vi "Teleop.vi"(10 "Match Info":T2={"Autonomous Elapsed Seconds"=0.0, "TeleOp Elapsed Seconds"=0.0, "Disabled Elapsed Seconds"=0.0, "Visited Autonomous"=FALSE, "Visited TeleOp"=FALSE, "Visited Disabled"=FALSE, "Autonomous Settings"={"Autonomous Style"=enum."Independent", "VI Refnum"=refnum}}, 11 "Call Context":T3) -> ()   [LabVIEW 2012]
doc: "This VI is called for each TeleOp packet received from the DS where the robot is not disabled. It is often used to read from the joysticks and update I/O or to update setpoints for timed control loops. It should complete and return within 20 milliseconds or it may miss DS packets."
uses:
  <vilib>/Rock Robotics/WPI/DriverStation/WPI_DriverStationDerivedRobotMode.ctl
  <vilib>/Rock Robotics/WPI/DriverStation/WPI_DriverStationMatch Info.ctl
  <vilib>/Rock Robotics/WPI/Relay/WPI_RelayValue.ctl
  <vilib>/Rock Robotics/WPI/Solenoid/WPI_SolenoidValue.ctl
  Robot Global Data.vi
  <vilib>/addons/control/pid/pid.llb/PID (DBL).vi
  <vilib>/Rock Robotics/WPI/RobotDrive/WPI_RobotDriveGetSetRefNum.vi
  <vilib>/Rock Robotics/WPI/Joystick/WPI_JoystickGetSetRefNum.vi
  <vilib>/Rock Robotics/WPI/Solenoid/WPI_SolenoidSetEnum.vi
  <vilib>/addons/control/pid/NI_PID_pid.lvlib
panel:
  in  "Boolean":bool
  in  "Time to twitch":dbl=1300.0
  in  "Time of start twitch":dbl
  in  "Turn speed for twitch":dbl=0.7
  in  "Twitch":string="Nope"
  in  "Threshold for shooter":dbl=0.015
  in  "Posistioned":string="Nothing"
  in  "Angle Target":dbl
  out "Distance From Target":dbl
  out "Ready To Fire":bool
  in  "S Off Time":dbl=1.2
  in  "S On Time":dbl=0.2
  in  "Time Last Fired":dbl
  in  "Current Status":string="Roaming"
  in  "Shooter Speed":dbl format="%.2f"
  in  "Shooter On":bool=TRUE
  out "Waveform Chart":cluster{"Rate":dbl, "Rate":dbl}(graph)
  out "Rate 1":dbl
  out "Rate 2":dbl
  in  "PID gains":T1={"proportional gain (Kc)"=1.0, "integral time (Ti, min)"=0.007, "derivative time (Td, min)"=0.0} {"derivative time (Td, min)" format="%.3f"; "integral time (Ti, min)" format="%.3f"; "proportional gain (Kc)" format="%.3f"}
  in  "Maximum Encoder speed":dbl=25000.0
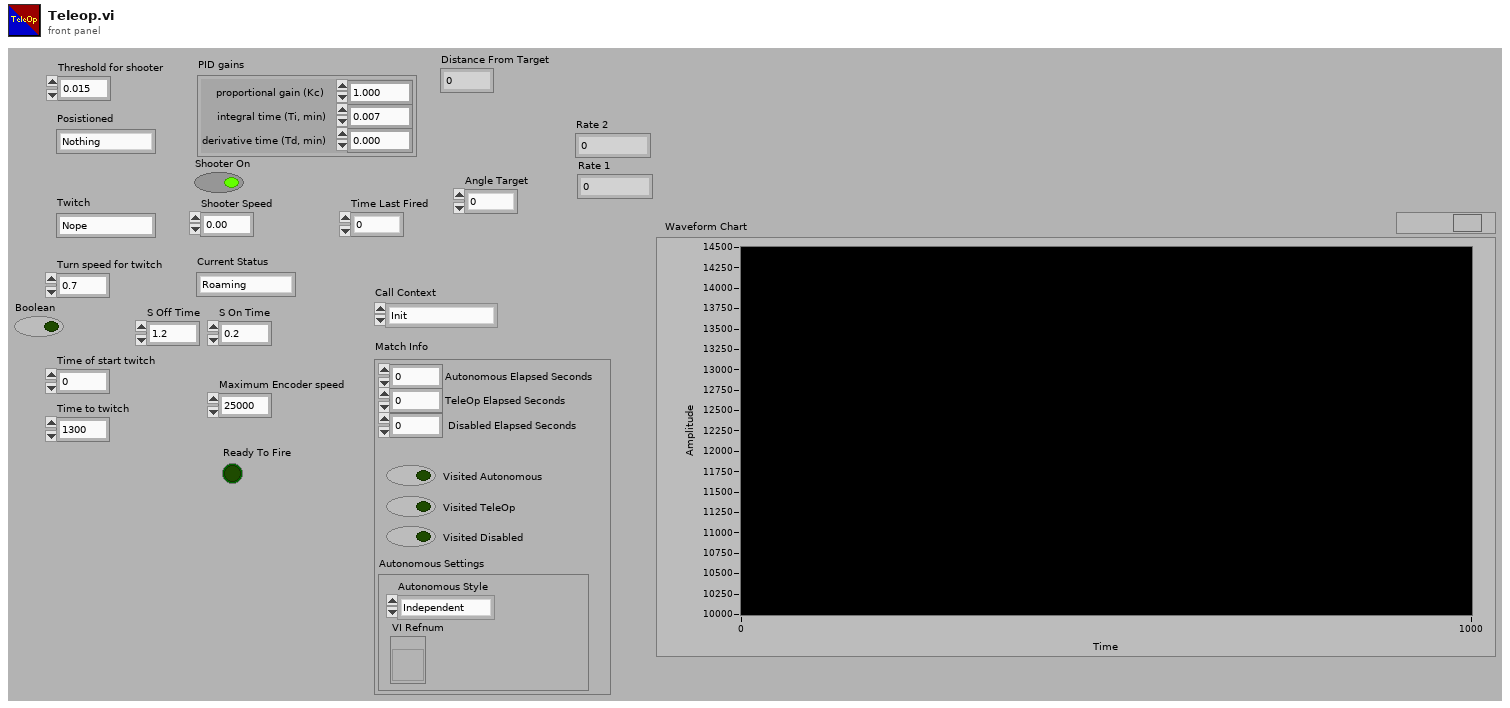
[diagram p1: front panel]
types:
  T1 = cluster{"proportional gain (Kc)":dbl, "integral time (Ti, min)":dbl, "derivative time (Td, min)":dbl}
  T2 = typedef "WPI_DriverStationMatch Info.ctl" = cluster{"Autonomous Elapsed Seconds":dbl, "TeleOp Elapsed Seconds":dbl, "Disabled Elapsed Seconds":dbl, "Visited Autonomous":bool, "Visited TeleOp":bool, "Visited Disabled":bool, "Autonomous Settings":cluster{"Autonomous Style":enum16{"Iterative", "Independent"}, "VI Refnum":refnum<vi>}}
  T3 = typedef "WPI_DriverStationDerivedRobotMode.ctl" = enum16{"Init", "Execute", "Stop"}
  T4 = typedef "WPI_EncoderDevRef.ctl" = cluster{"DevStatus":errorcluster, "EncoderIndex":T5, "CounterIndex":T6, "DistancePerCount":dbl, "Decoding Type":T7}
  T5 = typedef "FPGA_EncoderIdx.ctl" = enum8{"Enc 0", "Enc 1", "Enc 2", "Enc 3", "Invalid"}
  T6 = typedef "FPGA_CounterCtrSystemIndex.ctl" = enum8{"Ctr 0", "Ctr 1", "Ctr 2", "Ctr 3", "Ctr 4", "Ctr 5", "Ctr 6", "Ctr 7", "Invalid"}
  T7 = typedef "WPI_EncoderType.ctl" = enum16{"1x", "2x", "4x"}
  T8 = typedef "WPI_JoystickDevRef.ctl" = cluster{"Device":T9}
  T9 = typedef "WPI_JoystickDeviceEnum.ctl" = enum16{"USB 1", "USB 2", "USB 3", "USB 4", "Kinect 1", "Kinect 2"}
  T10 = typedef "WPI_JoystickButtonState.ctl" = cluster{"Button 1":bool, "Button 2":bool, "Button 3":bool, "Button 4":bool, "Button 5":bool, "Button 6":bool, "Button 7":bool, "Button 8":bool, "Button 9":bool, "Button 10":bool, "Button 11":bool, "Button 12":bool}
  T11 = cluster{"axis 1 (x)":dbl, "axis 2 (y)":dbl, "axis 3 (throttle)":dbl, "axis 4":dbl, "axis 5":dbl, "axis 6":dbl}
  T12 = typedef "WPI_RobotDriveDevRef.ctl" = cluster{"DevStatus":errorcluster, "Motors[]":T13[], "Square Inputs":bool, "Max Output":dbl, "Isochronous":bool}
  T13 = typedef "WPI_MotorControlDeviceRef.ctl" = cluster{"DeviceStatus":errorcluster, "Type":enum16{"PWM", "CAN"}, "PWM":cluster{"Digital Module":T14, "PWM Channel":T15, "DeadBand":T16}, "CAN":cluster{"Device Number":u8, "Control Mode":T17, "Semaphore":T18, "Max Vout":dbl}, "Invert":bool, "TransformRef":T19, "InvTransformRef":T19}
  T14 = typedef "FPGA_TypedefDigitalModule.ctl" = enum16{"Digital Module 1", "Digital Module 2"}
  T15 = typedef "FPGA_DIOPWMChannel.ctl" = enum8{"PWM 1", "PWM 2", "PWM 3", "PWM 4", "PWM 5", "PWM 6", "PWM 7", "PWM 8", "PWM 9", "PWM 10", "Invalid"}
  T16 = typedef "WPI_PWMDeadband.ctl" = cluster{"Name":string, "maxPositivePwm":i32, "minPositivePwm":i32, "centerPwm":i32, "maxNegativePwm":i32, "minNegativePwm":i32, "angularRange":u16}
  T17 = typedef "WPI_CANJaguar_ControlMode.ctl" = enum8{"Percent VBus", "Current", "Speed", "Position", "Voltage"}
  T18 = typedef "Semaphore RefNum" = refnum<k1>
  T19 = typedef "WPI_PWMTransform_ConPane.ctl" = refnum<vi>
  T20 = typedef "WPI_RelayValue.ctl" = enum16{"Off", "On", "Forward", "Reverse"}
  T21 = typedef "WPI_RelayDevRef.ctl" = cluster{"DevStatus":errorcluster, "Relay Channel":T22, "Digital Module":T14, "Relay Direction":T23}
  T22 = typedef "FPGA_DIORelayChannel.ctl" = enum8{"Relay 1", "Relay 2", "Relay 3", "Relay 4", "Relay 5", "Relay 6", "Relay 7", "Relay 8", "Invalid"}
  T23 = typedef "WPI_RelayDirection.ctl" = enum16{"Both directions", "Forward only", "Reverse only"}
  T24 = typedef "WPI_SolenoidValue.ctl" = enum16{"Off", "On", "Forward", "Reverse"}
  T25 = typedef "WPI_SolenoidDevRef.ctl" = cluster{"DevStatus":errorcluster, "Solenoid Module":T26, "Forward Solenoid Channel":T27, "Reverse Solenoid Channel":T27}
  T26 = typedef "FPGA_TypedefSolenoidModule.ctl" = enum16{"Solenoid Module 1", "Solenoid Module 2"}
  T27 = typedef "WPI_SolenoidChannel.ctl" = enum8{"Solenoid 1", "Solenoid 2", "Solenoid 3", "Solenoid 4", "Solenoid 5", "Solenoid 6", "Solenoid 7", "Solenoid 8", "Invalid"}
  T28 = cluster{"Center Position":cluster{"X":dbl, "Y":dbl}, "Distance (ft)":dbl, "Center":bool}[]
  T29 = cluster{"Center Position":cluster{"X":dbl, "Y":dbl}, "Distance (ft)":dbl, "Center":bool}
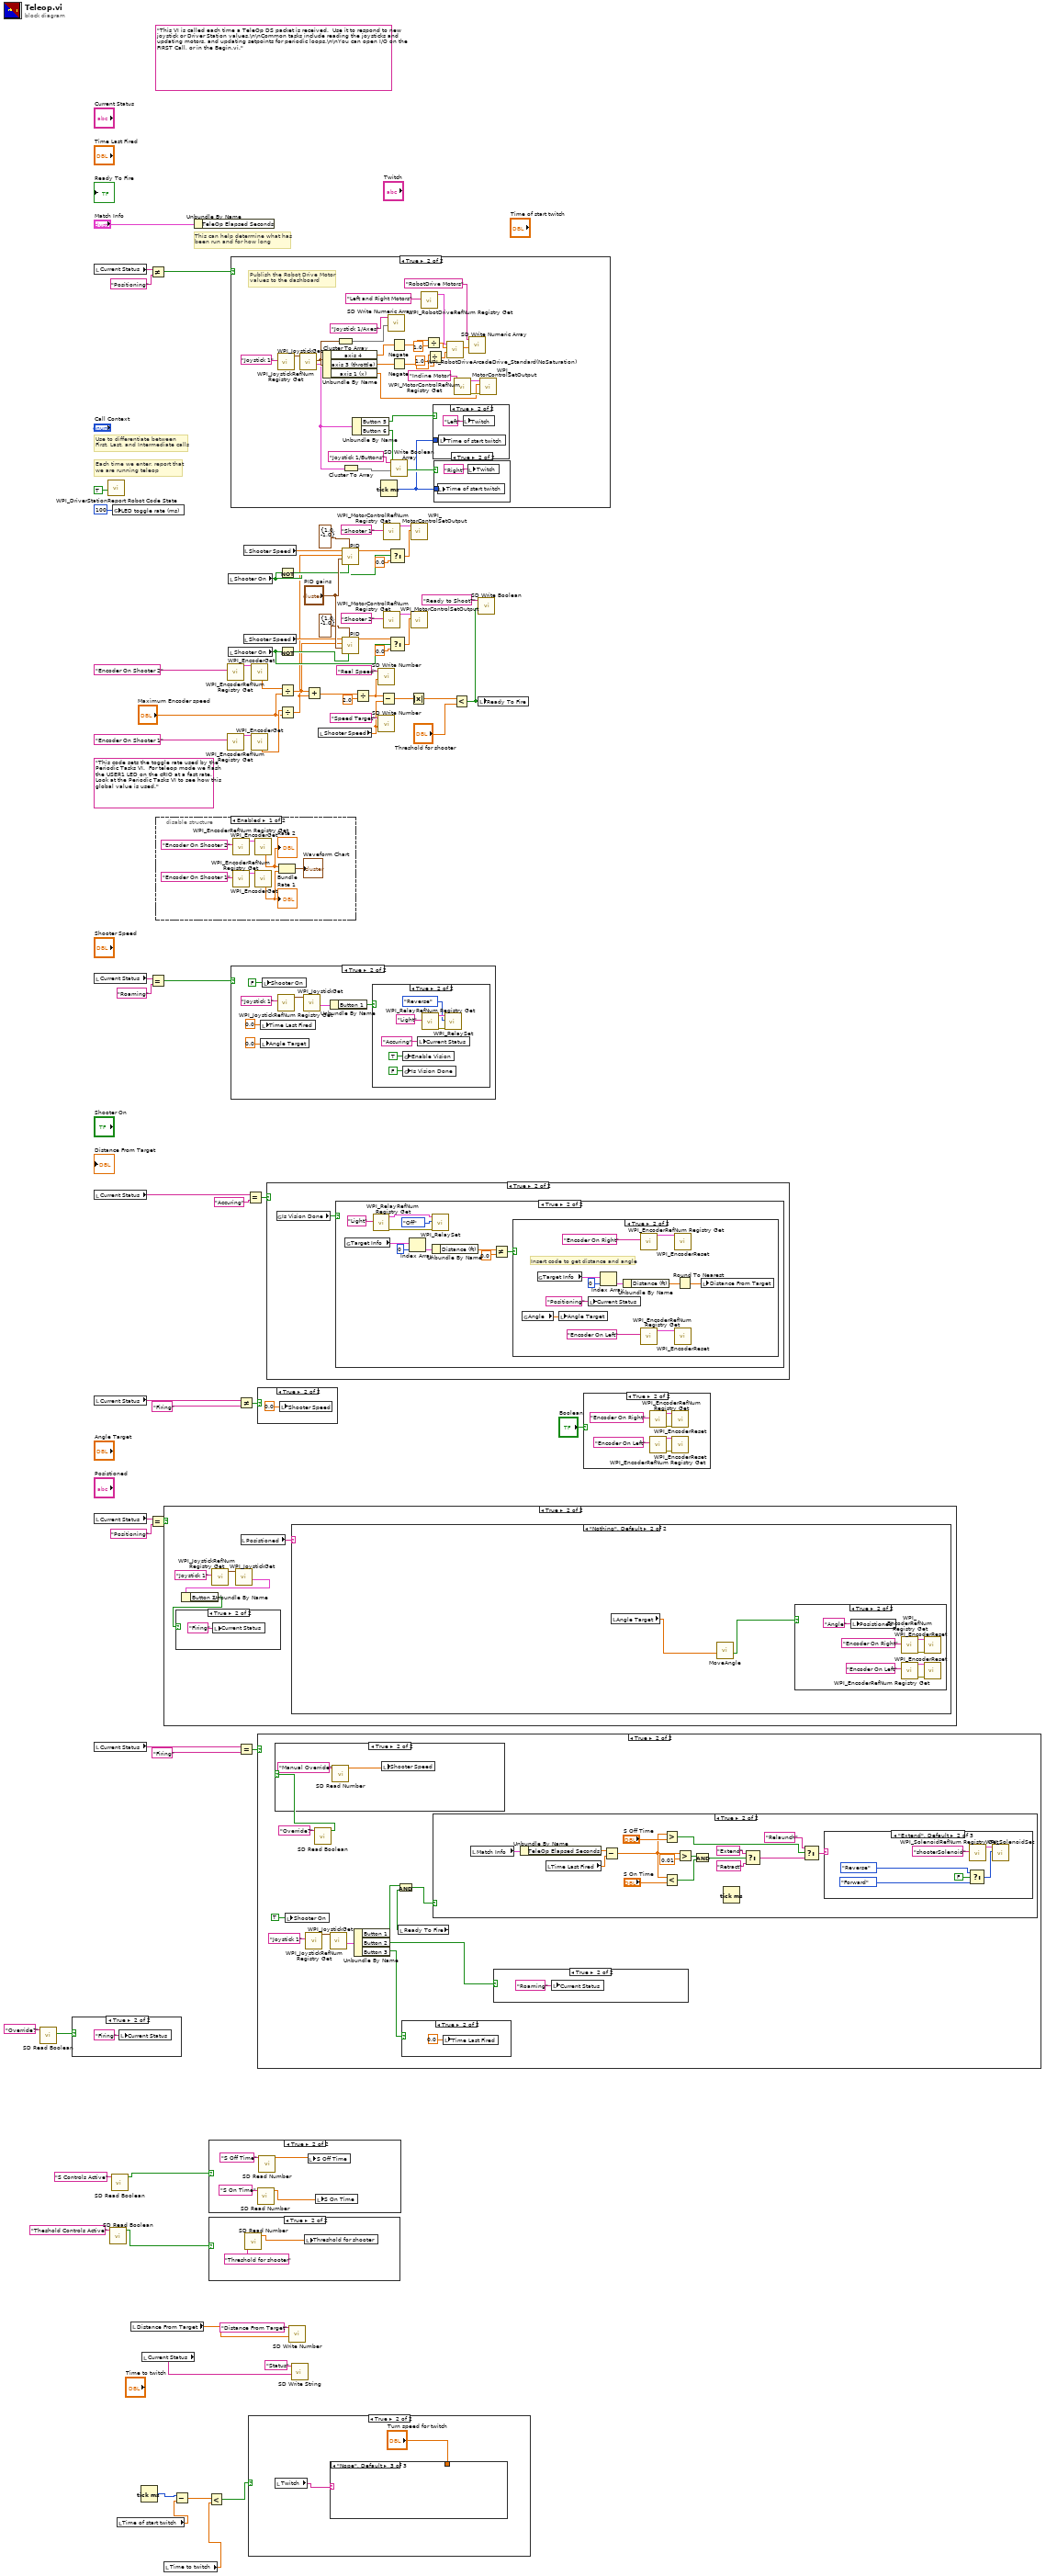
[diagram p0: block diagram]
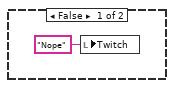
[diagram p3: hidden frame]
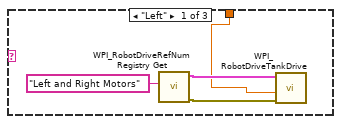
[diagram p4: hidden frame]
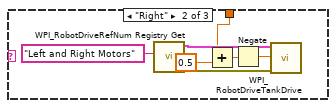
[diagram p5: hidden frame]
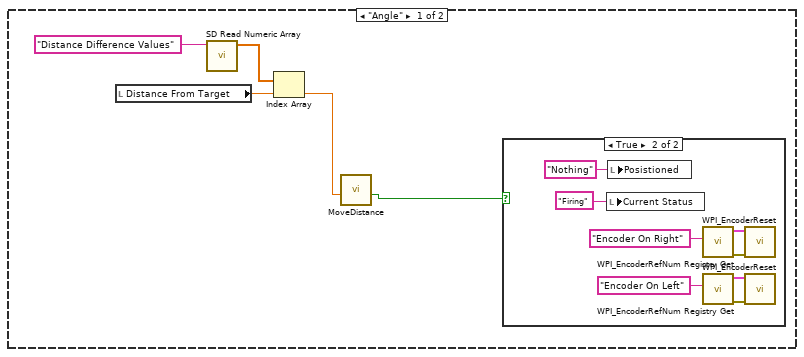
[diagram p12: hidden frame]
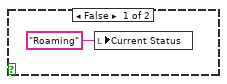
[diagram p20: hidden frame]
diagram:
  (unwired) "This code sets the toggle rate used by the Periodic Tasks VI.  For teleop mode we flash the USER1 LED on the cRIO at a fast rate.  Look at the Periodic Tasks VI to see how this global value is used."
  (unwired) "This VI is called each time a TeleOp DS packet is received.  Use it to respond to new joystick or Driver Station values.\n\nCommon tasks include reading the joysticks and updating motors, and updating setpoints for periodic loops.\n\nYou can open I/O on the FIRST Call, or in the Begin.vi."
  # "Each time we enter, report that\nwe are running teleop"
  # "Use to differentiate between\nFirst, Last, and Intermediate calls"
  # "This can help determine what has\nbeen run and for how long"
  n1 = call <vilib>:"SD Read Boolean.vi"("Name"="Override?") -> ("Boolean"=w15:bool)  [unwired: 8 in, 2 out]
  n2 = case shown="True" w15 {
    frame False {
    }
    frame True {
      n3 = local write "Current Status"("Firing" ("Current Status")) -> ()
    }
  }
  n4 = local read "Current Status"() -> (w26:string)
  n5 = local read "Current Status"() -> (w32:string)
  n6 = local read "Current Status"() -> (w29:string)
  n7 = local read "Current Status"() -> (w19:string)
  n8 = local read "Current Status"() -> (w23:string)
  n9 = local read "Current Status"() -> (w47:string)
  n10 = call <vilib>:"WPI_DriverStationReport Robot Code State.vi"("TeleOp"=TRUE ("Autonomous")) -> ()  [unwired: 10 in, 1 out]
  n11 = call <vilib>:"SD Read Boolean.vi"("Name"="Theshold Controls Active") -> ("Boolean"=w14:bool)  [unwired: 8 in, 2 out]
  n12 = call <vilib>:"SD Read Boolean.vi"("Name"="S Controls Active") -> ("Boolean"=w12:bool)  [unwired: 8 in, 2 out]
  n13 = global write "Robot Global Data.vi" "LED toggle rate (ms)"(u32 100 ("LED ms toggle rate")) -> ()
  n14 = local read "Time of start twitch"() -> (w6:dbl)
  n15 = local read "Distance From Target"() -> (w9:dbl)
  n16 = Tick Count (ms)() -> (millisecond timer value=w7:u32)
  n17 = local read "Current Status"() -> (w1:string)
  n18 = Not Equal?(x=w26, y="Positioning") -> (x != y?=w24:bool)
  n19 = Equal?(x=w32, y="Roaming") -> (x = y?=w30:bool)
  n20 = Equal?(x=w23, y="Positioning") -> (x = y?=w21:bool)
  n21 = disable-structure shown="Enabled" {
    frame Enabled {
      n22 = call <vilib>:"WPI_EncoderRefNum Registry Get.vi"("refnum name"="Encoder On Shooter 2") -> ("EncoderDevRef"=w83:T4)  [unwired: 9 in, 1 out]
      n23 = call <vilib>:"WPI_EncoderRefNum Registry Get.vi"("refnum name"="Encoder On Shooter 1") -> ("EncoderDevRef"=w82:T4)  [unwired: 9 in, 1 out]
      n24 = call <vilib>:"WPI_EncoderGet.vi"("EncoderDevRef"=w83) -> ("Rate"=w80:dbl)  [unwired: 5 in, 5 out]
      "Rate 2" <- w80
      n25 = call <vilib>:"WPI_EncoderGet.vi"("EncoderDevRef"=w82) -> ("Rate"=w81:dbl)  [unwired: 5 in, 5 out]
      "Rate 1" <- w81
      n26 = Bundle("Rate"=w80, "Rate"=w81) -> (→"Waveform Chart":cluster{"Rate":dbl, "Rate":dbl})  [unwired: 1 in]
    }
    frame Disabled {
    }
  }
  n27 = case shown="True" w21 {
    frame False {
    }
    frame True {
      n28 = call <vilib>:"WPI_JoystickRefNum Registry Get.vi"("refnum name"="Joystick 1") -> ("JoystickDevRef"=w87:T8)  [unwired: 9 in, 1 out]
      n29 = call <vilib>:"WPI_JoystickGet.vi"("JoystickDevRef"=w87) -> ("Buttons"=w86:T10)  [unwired: 4 in, 2 out]
      n30 = Unbundle By Name(w86) -> ("Button 2"=w85:bool)
      n31 = case shown="True" w85 {
        frame False {
        }
        frame True {
          n32 = local write "Current Status"("Firing" ("Current Status")) -> ()
        }
      }
      n33 = local read "Posistioned"() -> (w89:string)
      n34 = case shown="\"Nothing\", Default" w89 {
        frame "Angle" {
          n35 = local read "Distance From Target"() -> (w93:dbl)
          n36 = call <vilib>:"SD Read Numeric Array.vi"("Name"="Distance Difference Values") -> ("Numeric Array"=w95:dbl[])  [unwired: 8 in, 2 out]
          n37 = Index Array(array=w95, index=w93) -> (element=w92:dbl)
          n38 = call "MoveDistance.vi"("Distance From Target"=w92) -> ("Done?"=w91:bool)  [unwired: 10 in]
          n39 = case shown="True" w91 {
            frame False {
            }
            frame True {
              n40 = local write "Current Status"("Firing" ("Current Status")) -> ()
              n41 = local write "Posistioned"("Nothing" ("Posistioned")) -> ()
              n42 = call <vilib>:"WPI_EncoderRefNum Registry Get.vi"("refnum name"="Encoder On Right") -> ("error out"=w101:errorcluster, "EncoderDevRef"=w102:T4)  [unwired: 9 in]
              n43 = call <vilib>:"WPI_EncoderRefNum Registry Get.vi"("refnum name"="Encoder On Left") -> ("error out"=w99:errorcluster, "EncoderDevRef"=w100:T4)  [unwired: 9 in]
              n44 = call <vilib>:"WPI_EncoderReset.vi"("error in (no error)"=w101, "EncoderDevRef"=w102) -> ()  [unwired: 8 in, 2 out]
              n45 = call <vilib>:"WPI_EncoderReset.vi"("error in (no error)"=w99, "EncoderDevRef"=w100) -> ()  [unwired: 8 in, 2 out]
            }
          }
        }
        frame "Nothing", Default {
          n46 = local read "Angle Target"() -> (w105:dbl)
          n47 = call "MoveAngle.vi"("Angle Target"=w105) -> ("Done?"=w104:bool)  [unwired: 10 in]
          n48 = case shown="True" w104 {
            frame False {
            }
            frame True {
              n49 = local write "Posistioned"("Angle" ("Posistioned")) -> ()
              n50 = call <vilib>:"WPI_EncoderRefNum Registry Get.vi"("refnum name"="Encoder On Right") -> ("error out"=w108:errorcluster, "EncoderDevRef"=w107:T4)  [unwired: 9 in]
              n51 = call <vilib>:"WPI_EncoderRefNum Registry Get.vi"("refnum name"="Encoder On Left") -> ("error out"=w110:errorcluster, "EncoderDevRef"=w109:T4)  [unwired: 9 in]
              n52 = call <vilib>:"WPI_EncoderReset.vi"("error in (no error)"=w108, "EncoderDevRef"=w107) -> ()  [unwired: 8 in, 2 out]
              n53 = call <vilib>:"WPI_EncoderReset.vi"("error in (no error)"=w110, "EncoderDevRef"=w109) -> ()  [unwired: 8 in, 2 out]
            }
          }
        }
      }
    }
  }
  n54 = local read "Time to twitch"() -> (w4:dbl)
  n55 = Subtract(x=w7, y=w6) -> (x-y=w5:dbl)
  n56 = Unbundle By Name("Match Info") -> ()  [unwired: 1 out]
  n57 = Less?(x=w5, y=w4) -> (x < y?=w3:bool)
  n58 = case shown="True" w12 {
    frame False {
    }
    frame True {
      n59 = call <vilib>:"SD Read Number.vi"("Name"="S On Time") -> ("Numeric"=w115:dbl)  [unwired: 8 in, 2 out]
      n60 = call <vilib>:"SD Read Number.vi"("Name"="S Off Time") -> ("Numeric"=w116:dbl)  [unwired: 8 in, 2 out]
      n61 = local write "S Off Time"(w116) -> ()
      n62 = local write "S On Time"(w115) -> ()
    }
  }
  n63 = case shown="True" w14 {
    frame False {
    }
    frame True {
      n64 = call <vilib>:"SD Read Number.vi"("Name"="Threshold for shooter") -> ("Numeric"=w117:dbl)  [unwired: 8 in, 2 out]
      n65 = local write "Threshold for shooter"(w117) -> ()
    }
  }
  n66 = call <vilib>:"WPI_EncoderRefNum Registry Get.vi"("refnum name"="Encoder On Shooter 2") -> ("EncoderDevRef"=w61:T4)  [unwired: 9 in, 1 out]
  n67 = call <vilib>:"WPI_EncoderRefNum Registry Get.vi"("refnum name"="Encoder On Shooter 1") -> ("EncoderDevRef"=w70:T4)  [unwired: 9 in, 1 out]
  n68 = local read "Shooter On"() -> (w50:bool)
  n69 = local read "Shooter On"() -> (w51:bool)
  n70 = case shown="True" w24 {
    frame False {
    }
    frame True {
      # "Publish the Robot Drive Motor\nvalues to the dashboard"
      n71 = call <vilib>:"WPI_JoystickRefNum Registry Get.vi"("refnum name"="Joystick 1") -> ("JoystickDevRef"=w138:T8)  [unwired: 1 in, 9 out]
      n72 = call <vilib>:"WPI_JoystickGet.vi"("JoystickDevRef"=w138) -> ("Buttons"=w125:T10, "Axes"=w141:T11)  [unwired: 1 in, 4 out]
      n73 = Unbundle By Name(w141) -> ("axis 4"=w134:dbl, "axis 3 (throttle)"=w133:dbl, "axis 1 (x)"=w126:dbl)
      n74 = Cluster To Array(cluster=w141) -> (array=w142:dbl[])
      n75 = Cluster To Array(cluster=w125) -> (array=w139:bool[])
      n76 = Unbundle By Name(w125) -> ("Button 5"=w124:bool, "Button 6"=w123:bool)
      n77 = Tick Count (ms)() -> (millisecond timer value=w122:u32)
      n78 = call <vilib>:"SD Write Numeric Array.vi"("Numeric Array"=w142, "Name"="Joystick 1/Axes") -> ()  [unwired: 8 in, 2 out]
      n79 = Negate(x=w134) -> (-x=w132:dbl)
      n80 = Negate(x=w133) -> (-x=w120:dbl)
      n81 = call <vilib>:"SD Write Boolean Array.vi"("Boolean Array"=w139, "Name"="Joystick 1/Buttons") -> ()  [unwired: 8 in, 2 out]
      n82 = call <vilib>:"WPI_RobotDriveRefNum Registry Get.vi"("refnum name"="Left and Right Motors") -> ("RobotDriveDevRef"=w137:T12)  [unwired: 1 in, 9 out]
      n83 = Divide(x=w132, y=1.0) -> (x/y=w130:dbl)
      n84 = Divide(x=w120, y=1.0) -> (x/y=w121:dbl)
      n85 = case shown="True" w124 {
        tunnel: w122 -> [_ w146]
        frame False {
        }
        frame True {
          n86 = local write "Time of start twitch"(w146) -> ()
          n87 = local write "Twitch"("Left" ("Twitch")) -> ()
        }
      }
      n88 = case shown="True" w123 {
        tunnel: w122 -> [_ w148]
        frame False {
        }
        frame True {
          n89 = local write "Time of start twitch"(w148) -> ()
          n90 = local write "Twitch"("Right" ("Twitch")) -> ()
        }
      }
      n91 = call <vilib>:"WPI_RobotDriveArcadeDrive_Standard(NoSaturation).vi"("Y axis value"=w121, "X axis value"=w130, "RobotDriveDevRef"=w137) -> ("Motor Values"=w145:dbl[])  [unwired: 1 in, 7 out]
      n92 = call <vilib>:"WPI_MotorControlRefNum Registry Get.vi"("refnum name"="Incline Motor") -> ("error out"=w128:errorcluster, "MotorControlDevRef"=w127:T13)  [unwired: 9 in]
      n93 = call <vilib>:"SD Write Numeric Array.vi"("Numeric Array"=w145, "Name"="RobotDrive Motors") -> ()  [unwired: 8 in, 2 out]
      n94 = call <vilib>:"WPI_MotorControlSetOutput.vi"("error in (no error)"=w128, "Output"=w126, "MotorControlDevRef"=w127) -> ()  [unwired: 6 in, 3 out]
    }
  }
  n95 = case shown="True" w30 {
    frame False {
    }
    frame True {
      n96 = local write "Time Last Fired"(0.0 ("Time Last Fired")) -> ()
      n97 = local write "Angle Target"(0.0 ("Angle Target")) -> ()
      n98 = local write "Shooter On"(FALSE ("Shooter On")) -> ()
      n99 = call <vilib>:"WPI_JoystickRefNum Registry Get.vi"("refnum name"="Joystick 1") -> ("JoystickDevRef"=w155:T8)  [unwired: 9 in, 1 out]
      n100 = call <vilib>:"WPI_JoystickGet.vi"("JoystickDevRef"=w155) -> ("Buttons"=w154:T10)  [unwired: 4 in, 2 out]
      n101 = Unbundle By Name(w154) -> ("Button 1"=w153:bool)
      n102 = case shown="True" w153 {
        frame False {
        }
        frame True {
          n103 = global write "Robot Global Data.vi" "Enable Vision"(TRUE ("Enable Vision")) -> ()
          n104 = global write "Robot Global Data.vi" "Is Vision Done"(FALSE ("Is Vision Done")) -> ()
          n105 = local write "Current Status"("Accuring" ("Current Status")) -> ()
          n106 = call <vilib>:"WPI_RelayRefNum Registry Get.vi"("refnum name"="Light") -> ("error out"=w159:errorcluster, "RelayDevRef"=w160:T21)  [unwired: 9 in]
          n107 = call <vilib>:"WPI_RelaySet.vi"("error in (no error)"=w159, "RelayValue"=WPI_RelayValue."Reverse", "RelayDevRef"=w160) -> ()  [unwired: 7 in, 2 out]
        }
      }
    }
  }
  n108 = Not Equal?(x=w19, y="Firing") -> (x != y?=w18:bool)
  n109 = Equal?(x=w47, y="Firing") -> (x = y?=w45:bool)
  n110 = local read "Shooter Speed"() -> (w49:dbl)
  n111 = local read "Shooter Speed"() -> (w48:dbl)
  n112 = Equal?(x=w29, y="Accuring") -> (x = y?=w27:bool)
  n113 = case shown="True" w3 {
    frame False {
      n114 = local write "Twitch"("Nope" ("Twitch")) -> ()
    }
    frame True {
      n115 = local read "Twitch"() -> (w165:string)
      n116 = case shown="\"Nope\", Default" w165 {
        tunnel: "Turn speed for twitch" -> [w167 w173 _]
        frame "Left" {
          n117 = call <vilib>:"WPI_RobotDriveRefNum Registry Get.vi"("refnum name"="Left and Right Motors") -> ("error out"=w170:errorcluster, "RobotDriveDevRef"=w169:T12)  [unwired: 9 in]
          n118 = call <vilib>:"WPI_RobotDriveTankDrive.vi"("error in (no error)"=w170, "Right axis value"=w167, "RobotDriveDevRef"=w169) -> ()  [unwired: 6 in, 3 out]
        }
        frame "Right" {
          n119 = call <vilib>:"WPI_RobotDriveRefNum Registry Get.vi"("refnum name"="Left and Right Motors") -> ("error out"=w177:errorcluster, "RobotDriveDevRef"=w176:T12)  [unwired: 9 in]
          n120 = Add(x=w173, y=0.5) -> (x+y=w171:dbl)
          n121 = Negate(x=w171) -> (-x=w174:dbl)
          n122 = call <vilib>:"WPI_RobotDriveTankDrive.vi"("error in (no error)"=w177, "Left axis value"=w174, "RobotDriveDevRef"=w176) -> ()  [unwired: 6 in, 3 out]
        }
        frame "Nope", Default {
        }
      }
    }
  }
  n123 = call <vilib>:"WPI_EncoderGet.vi"("EncoderDevRef"=w61) -> ("Rate"=w53:dbl)  [unwired: 5 in, 5 out]
  n124 = call <vilib>:"WPI_EncoderGet.vi"("EncoderDevRef"=w70) -> ("Rate"=w54:dbl)  [unwired: 5 in, 5 out]
  n125 = case shown="True" w18 {
    frame False {
    }
    frame True {
      n126 = local write "Shooter Speed"(0.0 ("Shooter Speed")) -> ()
    }
  }
  n127 = case shown="True" w45 {
    frame False {
    }
    frame True {
      n128 = local write "Shooter On"(TRUE ("Shooter On")) -> ()
      n129 = call <vilib>:"WPI_JoystickRefNum Registry Get.vi"("refnum name"="Joystick 1") -> ("JoystickDevRef"=w188:T8)  [unwired: 9 in, 1 out]
      n130 = call <vilib>:"SD Read Boolean.vi"("Name"="Override?") -> ("Boolean"=w179:bool)  [unwired: 8 in, 2 out]
      n131 = case shown="True" w179 {
        frame False {
          n132 = local read "Distance From Target"() -> (w190:dbl)
          n133 = call <vilib>:"SD Read Numeric Array.vi"("Name"="Speed Values") -> ("Numeric Array"=w192:dbl[])  [unwired: 8 in, 2 out]
          n134 = Index Array(array=w192, index=w190) -> (element=w191:dbl)
          n135 = local write "Shooter Speed"(w191) -> ()
        }
        frame True {
          n136 = call <vilib>:"SD Read Number.vi"("Name"="Manual Override") -> ("Numeric"=w194:dbl)  [unwired: 8 in, 2 out]
          n137 = local write "Shooter Speed"(w194) -> ()
        }
      }
      n138 = call <vilib>:"WPI_JoystickGet.vi"("JoystickDevRef"=w188) -> ("Buttons"=w187:T10)  [unwired: 4 in, 2 out]
      n139 = Unbundle By Name(w187) -> ("Button 1"=w186:bool, "Button 2"=w182:bool, "Button 3"=w181:bool)
      n140 = local read "Ready To Fire"() -> (w184:bool)
      n141 = And(x=w186, y=w184) -> (x .and. y?=w185:bool)
      n142 = case shown="True" w181 {
        frame False {
        }
        frame True {
          n143 = local write "Time Last Fired"(0.0 ("Time Last Fired")) -> ()
        }
      }
      n144 = case shown="True" w185 {
        frame False {
        }
        frame True {
          n145 = local read "Match Info"() -> (w213:T2)
          n146 = Unbundle By Name(w213) -> ("TeleOp Elapsed Seconds"=w212:dbl)
          n147 = local read "Time Last Fired"() -> (w211:dbl)
          n148 = Subtract(x=w212, y=w211) -> (x-y=w204:dbl)
          n149 = Greater?(x=w204, y="S Off Time") -> (0:w207:bool)
          n150 = Less?(x=w204, y="S On Time") -> (x < y?=w201:bool)
          n151 = Greater?(x=w204, y=0.01) -> (0:w202:bool)
          n152 = And(x=w202, y=w201) -> (x .and. y?=w200:bool)
          n153 = Tick Count (ms)() -> ()  [unwired: 1 out]
          n154 = Select(t="Extend" ("f"), s=w200, f="Retract") -> (s? t:f=w205:string)
          n155 = Select(t="Relaunch" ("f"), s=w207, f=w205) -> (s? t:f=w209:string)
          n156 = case shown="\"Extend\", Default" w209 {
            frame "Retract" {
              n157 = Select(t=WPI_SolenoidValue."Reverse" ("Value"), s=TRUE, f=WPI_SolenoidValue."Forward" ("Value")) -> (s? t:f=w218:T24)
              n158 = call <vilib>:"WPI_SolenoidRefNum Registry Get.vi"("refnum name"="shooterSolenoid") -> ("SolenoidDevRef"=w214:T25)  [unwired: 9 in, 1 out]
              n159 = call-poly <vilib>:"WPI_SolenoidSet.vi"("Value"=w218, "SolenoidDevRef"=w214) -> ()  [unwired: 8 in, 2 out]
            }
            frame "Extend", Default {
              n160 = Select(t=WPI_SolenoidValue."Reverse" ("Value"), s=FALSE, f=WPI_SolenoidValue."Forward" ("Value")) -> (s? t:f=w224:T24)
              n161 = call <vilib>:"WPI_SolenoidRefNum Registry Get.vi"("refnum name"="shooterSolenoid") -> ("SolenoidDevRef"=w220:T25)  [unwired: 9 in, 1 out]
              n162 = call-poly <vilib>:"WPI_SolenoidSet.vi"("Value"=w224, "SolenoidDevRef"=w220) -> ()  [unwired: 8 in, 2 out]
            }
            frame "Relaunch" {
              n163 = local read "Match Info"() -> (w227:T2)
              n164 = Unbundle By Name(w227) -> ("TeleOp Elapsed Seconds"=w226:dbl)
              n165 = local write "Time Last Fired"(w226) -> ()
            }
          }
        }
      }
      n166 = case shown="True" w182 {
        frame False {
        }
        frame True {
          n167 = local write "Current Status"("Roaming" ("Current Status")) -> ()
        }
      }
    }
  }
  n168 = case shown="True" w27 {
    frame False {
    }
    frame True {
      n169 = global read "Robot Global Data.vi" "Is Vision Done"() -> (w228:bool)
      n170 = case shown="True" w228 {
        frame False {
        }
        frame True {
          n171 = global read "Robot Global Data.vi" "Target Info"() -> (w238:T28)
          n172 = call <vilib>:"WPI_RelayRefNum Registry Get.vi"("refnum name"="Light") -> ("error out"=w231:errorcluster, "RelayDevRef"=w232:T21)  [unwired: 9 in]
          n173 = Index Array(array=w238, index=0) -> (element=w236:T29)
          n174 = call <vilib>:"WPI_RelaySet.vi"("error in (no error)"=w231, "RelayValue"=WPI_RelayValue."Off", "RelayDevRef"=w232) -> ()  [unwired: 7 in, 2 out]
          n175 = Unbundle By Name(w236) -> ("Distance (ft)"=w234:dbl)
          n176 = Not Equal?(x=w234, y=0.0) -> (x != y?=w235:bool)
          n177 = case shown="True" w235 {
            frame False {
              n178 = local write "Current Status"("Roaming" ("Current Status")) -> ()
            }
            frame True {
              # "Insert code to get distance and angle"
              n179 = global read "Robot Global Data.vi" "Angle"() -> (w245:dbl)
              n180 = global read "Robot Global Data.vi" "Target Info"() -> (w244:T28)
              n181 = local write "Angle Target"(w245) -> ()
              n182 = local write "Current Status"("Positioning" ("Current Status")) -> ()
              n183 = Index Array(array=w244, index=0) -> (element=w242:T29)
              n184 = Unbundle By Name(w242) -> ("Distance (ft)"=w241:dbl)
              n185 = call <vilib>:"WPI_EncoderRefNum Registry Get.vi"("refnum name"="Encoder On Right") -> ("EncoderDevRef"=w247:T4)  [unwired: 9 in, 1 out]
              n186 = call <vilib>:"WPI_EncoderRefNum Registry Get.vi"("refnum name"="Encoder On Left") -> ("EncoderDevRef"=w248:T4)  [unwired: 9 in, 1 out]
              n187 = call <vilib>:"WPI_EncoderReset.vi"("EncoderDevRef"=w247) -> ()  [unwired: 9 in, 2 out]
              n188 = call <vilib>:"WPI_EncoderReset.vi"("EncoderDevRef"=w248) -> ()  [unwired: 9 in, 2 out]
              n189 = Round To Nearest(number=w241) -> (nearest integer value=w240:dbl)
              n190 = local write "Distance From Target"(w240) -> ()
            }
          }
        }
      }
    }
  }
  n191 = Not(x=w50) -> (.not. x?=w72:bool)
  n192 = Not(x=w51) -> (.not. x?=w63:bool)
  n193 = Divide(x=w53, y="Maximum Encoder speed") -> (x/y=w43:dbl)
  n194 = Divide(x=w54, y="Maximum Encoder speed") -> (x/y=w42:dbl)
  n195 = call <vilib>:"SD Write Number.vi"("Numeric"=w9, "Name"="Distance From Target") -> ()  [unwired: 8 in, 2 out]
  n196 = call <vilib>:"SD Write String.vi"("String"=w1, "Name"="Status") -> ()  [unwired: 8 in, 2 out]
  n197 = Add(x=w43, y=w42) -> (x+y=w41:dbl)
  n198 = local read "Shooter Speed"() -> (w38:dbl)
  n199 = call-poly <vilib>:"PID.vi"("reinitialize? (F)"=w72, "output range"=cluster{"output high":dbl, "output low":dbl} {"output high"=1.0, "output low"=-1.0}, "PID gains"="PID gains", "process variable"=w42, "setpoint"=w49) -> ("output"=w71:dbl)  [unwired: 5 in, 1 out]
  n200 = call-poly <vilib>:"PID.vi"("reinitialize? (F)"=w63, "output range"=cluster{"output high":dbl, "output low":dbl} {"output high"=1.0, "output low"=-1.0}, "PID gains"="PID gains", "process variable"=w43, "setpoint"=w48) -> ("output"=w62:dbl)  [unwired: 5 in, 1 out]
  n201 = Divide(x=w41, y=2.0) -> (x/y=w37:dbl)
  n202 = call <vilib>:"SD Write Number.vi"("Numeric"=w37, "Name"="Real Speed") -> ()  [unwired: 8 in, 2 out]
  n203 = call <vilib>:"SD Write Number.vi"("Numeric"=w38, "Name"="Speed Target") -> ()  [unwired: 8 in, 2 out]
  n204 = Subtract(x=w37, y=w38) -> (x-y=w36:dbl)
  n205 = call <vilib>:"WPI_MotorControlRefNum Registry Get.vi"("refnum name"="Shooter 1") -> ("MotorControlDevRef"=w65:T13)  [unwired: 9 in, 1 out]
  n206 = call <vilib>:"WPI_MotorControlRefNum Registry Get.vi"("refnum name"="Shooter 2") -> ("MotorControlDevRef"=w56:T13)  [unwired: 9 in, 1 out]
  n207 = Select(t=w71, s=w50, f=0.0) -> (s? t:f=w67:dbl)
  n208 = Select(t=w62, s=w51, f=0.0) -> (s? t:f=w58:dbl)
  n209 = Absolute Value(x=w36) -> (abs(x)=w35:dbl)
  n210 = call <vilib>:"WPI_MotorControlSetOutput.vi"("Output"=w67, "MotorControlDevRef"=w65) -> ()  [unwired: 7 in, 3 out]
  n211 = call <vilib>:"WPI_MotorControlSetOutput.vi"("Output"=w58, "MotorControlDevRef"=w56) -> ()  [unwired: 7 in, 3 out]
  n212 = Less?(x=w35, y="Threshold for shooter") -> (x < y?=w33:bool)
  n213 = call <vilib>:"SD Write Boolean.vi"("Boolean"=w33, "Name"="Ready to Shoot?") -> ()  [unwired: 8 in, 2 out]
  n214 = local write "Ready To Fire"(w33) -> ()
  n215 = case shown="True" "Boolean" {
    frame False {
    }
    frame True {
      n216 = call <vilib>:"WPI_EncoderRefNum Registry Get.vi"("refnum name"="Encoder On Right") -> ("error out"=w255:errorcluster, "EncoderDevRef"=w256:T4)  [unwired: 9 in]
      n217 = call <vilib>:"WPI_EncoderRefNum Registry Get.vi"("refnum name"="Encoder On Left") -> ("error out"=w253:errorcluster, "EncoderDevRef"=w254:T4)  [unwired: 9 in]
      n218 = call <vilib>:"WPI_EncoderReset.vi"("error in (no error)"=w255, "EncoderDevRef"=w256) -> ()  [unwired: 8 in, 2 out]
      n219 = call <vilib>:"WPI_EncoderReset.vi"("error in (no error)"=w253, "EncoderDevRef"=w254) -> ()  [unwired: 8 in, 2 out]
    }
  }
